vi "MPM_Get_IPAddress.vi"(8 "error in (no error)":errorcluster, 11 ".NET Reference in":refnum<k24>) -> (0 "error out":errorcluster, 2 "address out":string, 3 "Reference out":refnum<k24>)   [LabVIEW 2017]
uses:
  D:/test/FULLband-sts/Fullband_Sample/DLL/InstrumentDLL.dll
  DLL/InstrumentDLL.dll
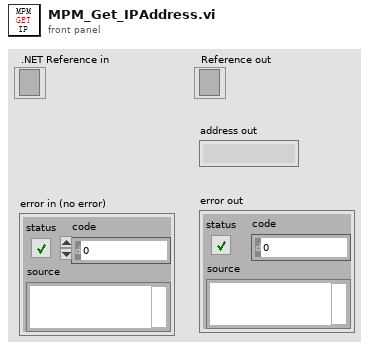
[diagram p1: front panel]
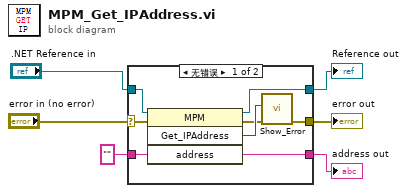
[diagram p0: block diagram]
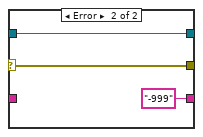
[diagram p2: hidden frame]
diagram:
  n1 = case shown="无错误" "error in (no error)" {
    selector: "error in (no error)" -> [w10 w16]
    tunnel: [w14 "-999" ("address")] -> w6
    tunnel: ".NET Reference in" -> [w13 w17]
    tunnel: [w12 w17] -> w4
    tunnel: "" ("address") -> [w11 _]
    tunnel: [w7 w16] -> w1
    frame No Error {
      n2 = invoke class="MPM" method="Get_IPAddress"(reference=w13, error in=w10, "address"=w11) -> (reference out=w12:refnum<k24>, error out=w8:errorcluster, "Get_IPAddress"=w9:i32, "address"=w14:string)  [unwired: 1 in]
      n3 = call "Show_Error.vi"("error in (no error)"=w8, "Error"=w9) -> ("error out"=w7:errorcluster)  [unwired: 9 in]
    }
    frame Error {
    }
  }
  "address out" <- w6
  "Reference out" <- w4
  "error out" <- w1
